vi "Move_Traverse_Client.vi"(4 "Speed Factor":dbl=1.0 min=0.1 max=5.0 format="%.2f", 5 "Backlash Compensation?":bool, 6 "Route Checking?":bool, 7 "Mode":T1=enum."Read traverse position", 8 "Traverse Position":dbl[](array[numeric])=[0.0, 0.0, 0.0] format="%.2f", 9 "Coordinate rotation (deg)":dbl format="%.2f", 10 "Traverse name":string) -> (0 "Error String":string, 2 "Position Acheived":dbl[](array[numeric]) format="%.2f")   [LabVIEW 2010]
doc: "This is an example of using features of the VI Server as a client. It shows how you might browse from one or more applications that may be exporting data from one or more data stations. \n\nThe example shows how to query a server for its list of exported VIs, how to get references to the VIs, and how call them with the Call By Reference function."
uses:
  Anemometry/Anemometry Sub Vis/Gen Trav/Trav_mode.ctl
  Anemometry/Anemometry Sub Vis/Globals/Constants_global.vi
  Anemometry/Anemometry Sub Vis/Globals/Meas_global.vi
  Anemometry/Anemometry Sub Vis/Globals/Trav_pos_global.vi
panel:
  in  "Traverse VI":refnum<vi>
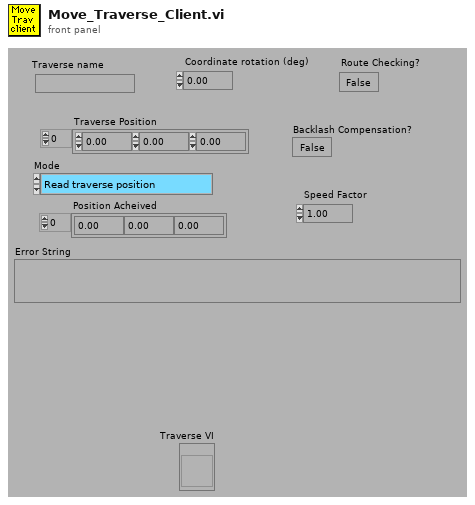
[diagram p1: front panel]
types:
  T1 = typedef "Trav_mode.ctl" = enum16{"Move traverse", "Read traverse position", "Teach Position"}
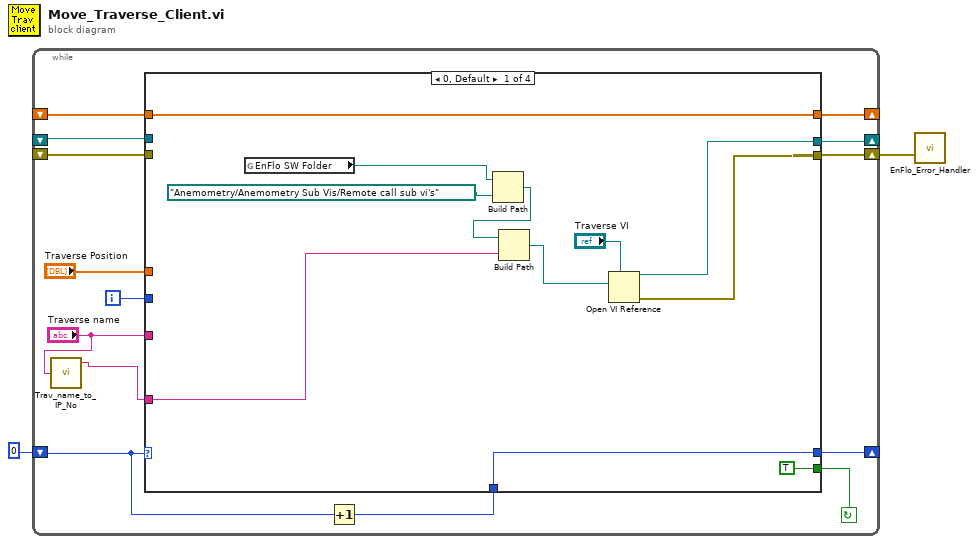
[diagram p0: block diagram]
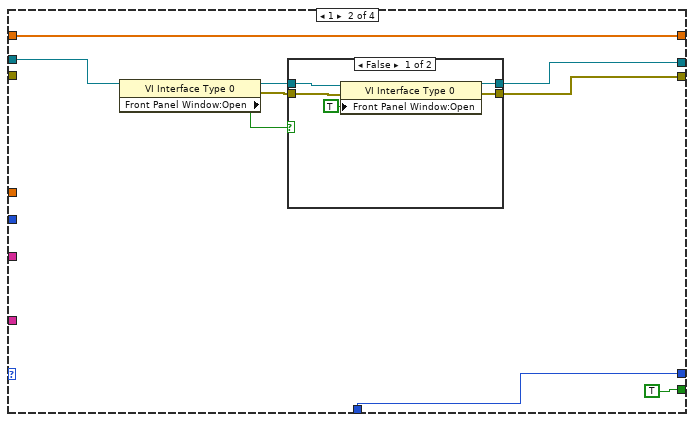
[diagram p2: hidden frame]
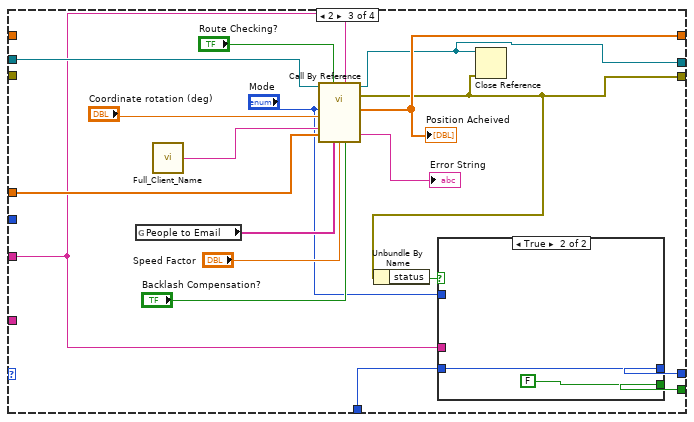
[diagram p4: hidden frame]
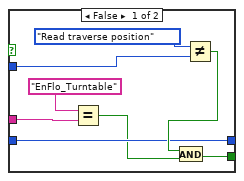
[diagram p5: hidden frame]
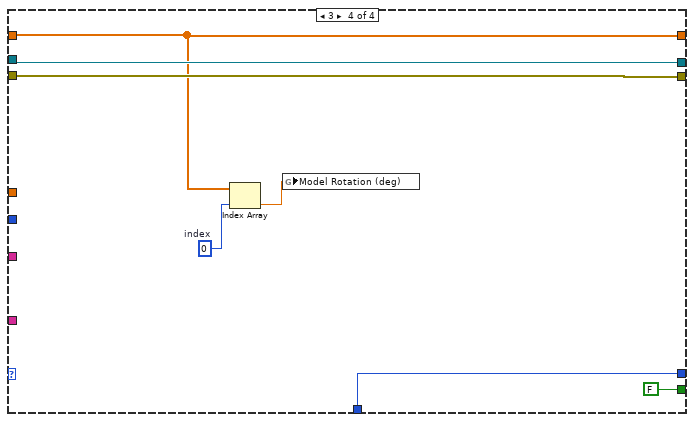
[diagram p6: hidden frame]
diagram:
  n1 = while {
    shift-left: 0 -> [w3]
    shift-right: [w10] -> _
    shift-left: _ -> [w16]
    shift-right: [w15] -> _
    shift-right: [w9] -> w1
    shift-left: _ -> [w8]
    shift-right: [w7] -> _
    shift-left: _ -> [w6]
    i -> [w14]
    stop <- w13 continue-if-true
    n2 = call "Trav_name_to_IP_No.vi"("Trav name"="Traverse name") -> ("VI name"=w5:string)  [unwired: 2 out]
    n3 = Increment(x=w3) -> (x+1=w11:i32)
    n4 = case shown="0, Default" w3 {
      tunnel: w16 -> [_ w36 w60 w78]
      tunnel: [w27 w32 w44 w78] -> w15
      tunnel: w14 -> [_ _ _ _]
      tunnel: [TRUE ("status") TRUE ("status") w49 FALSE ("status")] -> w13
      tunnel: "Traverse Position" -> [_ _ w58 _]
      tunnel: w5 -> [w18 _ _ _]
      tunnel: [w25 w31 w45 w77] -> w9
      tunnel: w11 -> [w24 w28 w51 w76]
      tunnel: [w24 w28 w50 w76] -> w10
      tunnel: w8 -> [_ _ _ w77]
      tunnel: [w23 w29 w47 w72] -> w7
      tunnel: w6 -> [w23 w29 _ w72]
      tunnel: "Traverse name" -> [_ _ w46 _]
      frame 0, Default {
        n5 = global read "Constants_global.vi" "EnFlo SW Folder"() -> (w22:path)
        n6 = Build Path(base path=w22, name or relative path=path "Anemometry/Anemometry Sub Vis/Remote call sub vi's") -> (appended path=w20:path)
        n7 = Build Path(base path=w20, name or relative path=w18) -> (appended path=w19:path)
        n8 = Open VI Reference(type specifier VI Refnum (for type only)="Traverse VI", vi path=w19) -> (vi reference=w27:refnum<vi>, error out=w25:errorcluster)  [unwired: 1 in, 3 out]
      }
      frame 1 {
        n9 = property class="VI Interface Type 0"(reference=w36) -> (reference out=w34:refnum<vi>, error out=w33:errorcluster, "Front Panel Window:Open"=w35:bool)  [unwired: 1 in]
        n10 = case shown="False" w35 {
          tunnel: w34 -> [w41 w43]
          tunnel: w33 -> [w40 w42]
          tunnel: [w39 w43] -> w32
          tunnel: [w38 w42] -> w31
          frame False {
            n11 = property class="VI Interface Type 0"(reference=w41, error in=w40, "Front Panel Window:Open"=TRUE) -> (reference out=w39:refnum<vi>, error out=w38:errorcluster)
          }
          frame True {
          }
        }
      }
      frame 2 {
        n12 = global read "Meas_global.vi" "People to Email"() -> (w59:string[])
        n13 = call "Full_Client_Name.vi"() -> ("Client Name"=w56:string)
        n14 = call-by-ref "?"(reference=w60, "Mode"="Mode", "Route Checking?"="Route Checking?", "Traverse Name"=w46, "Coordinate rotation (deg)"="Coordinate rotation (deg)", "Client's name"=w56, "Position input XYZ"=w58, "People to Email"=w59, "Speed Factor"="Speed Factor", "Backlash Compensation?"="Backlash Compensation?") -> (reference out=w44:refnum<vi>, error out=w45:errorcluster, "Position Output XYZ"=w47:dbl[], "Error String"=→"Error String":string)  [unwired: 6 in]
        "Position Acheived" <- w47
        n15 = Unbundle By Name(w45) -> ("status"=w52:bool)
        n16 = case shown="True" w52 {
          tunnel: w51 -> [w65 w70]
          tunnel: [w65 w70] -> w50
          tunnel: [w64 FALSE] -> w49
          tunnel: "Mode" -> [w68 _]
          tunnel: w46 -> [w63 _]
          frame False {
            n17 = Equal?(x="EnFlo_Turntable" ("y"), y=w63) -> (x = y?=w62:bool)
            n18 = Not Equal?(x=Trav_mode."Read traverse position" ("Mode"), y=w68) -> (x != y?=w66:bool)
            n19 = And(x=w66, y=w62) -> (x .and. y?=w64:bool)
          }
          frame True {
          }
        }
        n20 = Close Reference(reference=w44, error in (no error)=w45) -> ()  [unwired: 1 out]
      }
      frame 3 {
        w73 = 0  # index
        n21 = Index Array(array=w72, index=w73) -> (element=w74:dbl)
        n22 = global write "Trav_pos_global.vi" "Model Rotation (deg)"(w74) -> ()
      }
    }
  }
  n23 = call "EnFlo_Error_Handler.vi"("error in (no error)"=w1) -> ()  [unwired: 2 in, 3 out]
